vi "FilterFaulty.vi"(10 "Prev. Measurement In":dbl, 11 "Measurement In":dbl) -> (3 "Measurement Out":dbl)   [LabVIEW 2014]
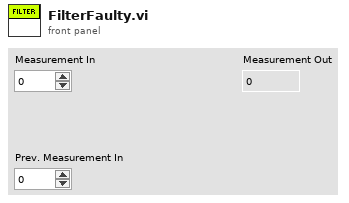
[diagram p1: front panel]
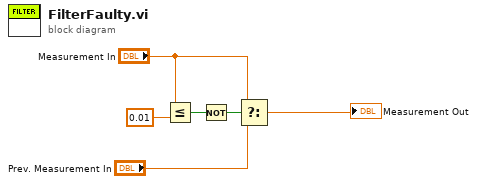
[diagram p0: block diagram]
diagram:
  n1 = Less Or Equal?(x="Measurement In", y=0.01) -> (x <= y?=w4:bool)
  n2 = Not(x=w4) -> (.not. x?=w5:bool)
  n3 = Select(t="Measurement In", s=w5, f="Prev. Measurement In") -> (s? t:f=→"Measurement Out":dbl)
